vi "Set Transceiver Options.vi"(8 "error in (no error)":errorcluster, 9 "Parameter":T1(ring), 11 "PPT in":refnum<class "PPT.lvclass">) -> (0 "error out":errorcluster, 3 "PPT out":refnum<class "PPT.lvclass">)   [LabVIEW 2014, in "PPT Library.lvlib" / "PPT.lvclass"]
doc: "Set the transceiver operating parameters. See PPT documentation to determine how the input parameter is applied."
uses:
  PPT.lvclass
  reusable/Session APIs/Serial/Serial Session.lvclass
  PPT.lvclass/PPT.ctl
  reusable/Session APIs/Serial/Public/Asynchronous Write.vi
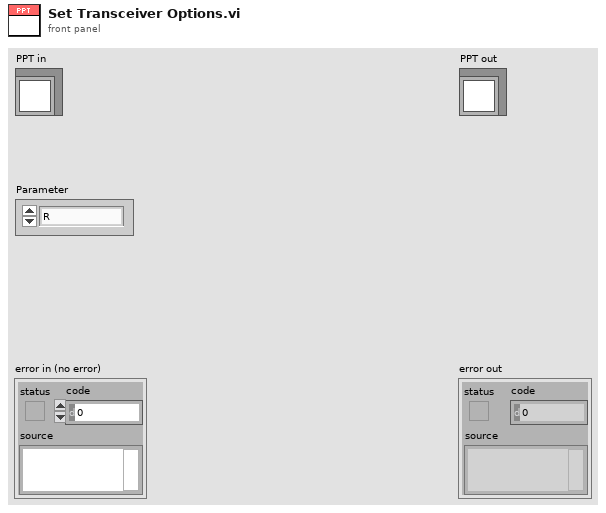
[diagram p1: front panel]
types:
  T1 = enum8{"R", "M", "C", "A", "S", "H", "0", "1", "2", "3", "N", "P"}
  T2 = typedef "Session - Root.lvclass/Session Handle.ctl" = refnum<data-value>
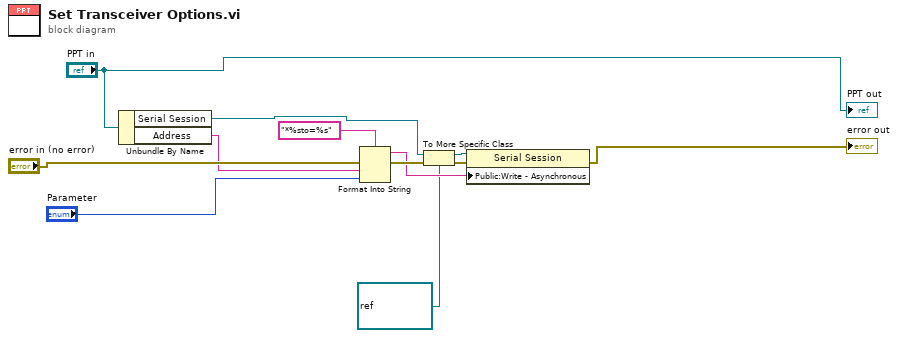
[diagram p0: block diagram]
diagram:
  n1 = Unbundle By Name("PPT in") -> ("Serial Session"=w3:T2, "Address"=w1:string)
  n2 = Format Into String(format string="*%sto=%s", error in="error in (no error)", w1, "Parameter") -> (resulting string=w4:string, error out=w5:errorcluster)  [unwired: 1 in]
  n3 = To More Specific Class(target class=refnum<data-value> refnum ("Serial Session"), reference=w3, error in=w5) -> (specific class reference=w8:refnum<data-value>, error out=w7:errorcluster)
  n4 = property class="Serial Session"(reference=w8, error in=w7, "Public:Write - Asynchronous"=w4) -> (error out=→"error out":errorcluster)  [unwired: 1 out]
  "PPT out" <- "PPT in"
